vi "Read Multiple Event Registration.vi"(11 "Test Case In":refnum<class "Tests Event MessengerM.lvclass">) -> (0 "error out":errorcluster, 3 "Test Case Out":refnum<class "Tests Event MessengerM.lvclass">)   [LabVIEW 2020, in "Tests Event MessengerM.lvclass"]
uses:
  Tests Event MessengerM.lvclass
  Tests Event MessengerM.lvclass/Tests Event MessengerM.ctl
  C:/Program Files/National Instruments/LabVIEW 2026/vi.lib/Astemes/LUnit/Test Case.lvclass
  C:/Program Files/National Instruments/LabVIEW 2026/vi.lib/Astemes/LUnit/LUnit Runnable.lvclass
  D:/git/Event-MessengerM-Channel-Wire/tests/Tests Event MessengerM/Tests Event MessengerM.lvclass
  <vilib>/Astemes/LUnit/Test Case.lvclass
  4a87e2e1-9280-4bda-9c4f-14fca454df33.vi
  66c5d38c-d599-4b3c-b5fe-0ff2804ba194.vi
  4a2384a7-b9c3-4d6f-8ce3-db5ad262e870.vi
  3cda7afb-27d7-4926-bd3c-22bc82fc3959.vi
  fb264298-76b7-4d75-ae4f-a2dcca52a52e.vi
panel:
  out "Array 2":string[](array[string])
  out "Array":string[](array[string])
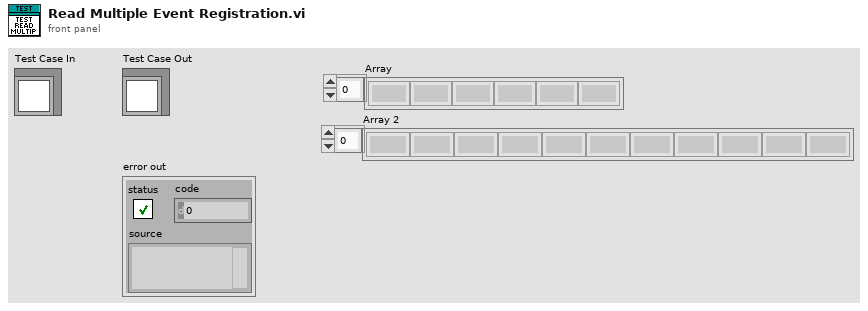
[diagram p1: front panel]
types:
  T1 = typedef "Event MessengerM-c(str,var).lvlib/))Channel.ctl" = refnum<queue>
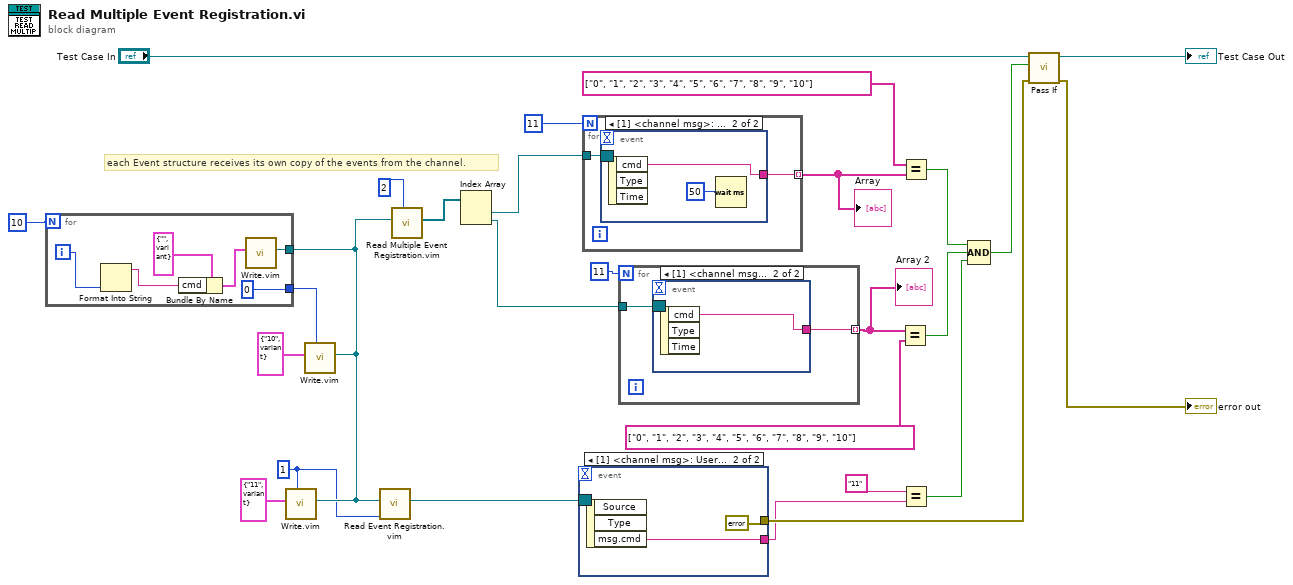
[diagram p0: block diagram]
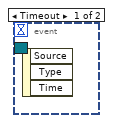
[diagram p2: hidden frame]
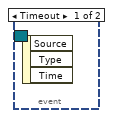
[diagram p3: hidden frame]
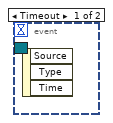
[diagram p4: hidden frame]
diagram:
  w2 = 1 ("subchannel (0)")
  # "each Event structure receives its own copy of the events from the channel."
  n1 = for {
    N: 10 -> [_]
    tunnel: [0] -> w7
    tunnel: [w28] -> w4
    i -> [w32]
    n2 = Format Into String(w32) -> (resulting string=w31:string)  [unwired: 3 in, 1 out]
    n3 = Bundle By Name(cluster=cluster{"cmd":string, "data":variant} {"cmd"="", "data"=variant} ("element"), "cmd"=w31) -> (w29:cluster{"cmd":string, "data":variant})
    n4 = call "Write.vim"("element"=w29) -> ("channel"=w28:T1)  [unwired: 9 in, 1 out]
  }
  n5 = call "Write.vim"("channel"=w4, "subchannel"=w2, "element"=cluster{"cmd":string, "data":variant} {"cmd"="11", "data"=variant}) -> ()  [unwired: 8 in, 1 out]
  n6 = call "Write.vim"("channel"=w4, "subchannel"=w7, "element"=cluster{"cmd":string, "data":variant} {"cmd"="10", "data"=variant}) -> ()  [unwired: 8 in, 1 out]
  n7 = call "Read Event Registration.vim"("subchannel"=w2, "channel"=w4) -> ("event registration refnum"=w5:refnum<event-registration>)  [unwired: 9 in]
  n8 = call "Read Multiple Event Registration.vim"("number of event structures"=u16 2, "channel in"=w4) -> ("event registration refnums"=w1:refnum<event-registration>[])  [unwired: 9 in]
  n9 = Index Array(array=w1) -> (element #1=w17:refnum<event-registration>, element #2=w16:refnum<event-registration>)  [unwired: 2 in]
  n10 = event shown="[1] <channel msg>: User Event" {
    selector: w5 -> [_ _]
    dyn-events: _ -> [_ _]
    timeout: _ -> [_ _]
    tunnel: [_ errorcluster {"status"=FALSE, "code"=0, "source"=""} ("error constant")] -> w18
    tunnel: [_ w34] -> w13
    event Timeout {
      n11 = event-data() -> ()  [unwired: 1 in, 3 out]
    }
    event User Event {
      n12 = event-data() -> ("msg.cmd"=w34:string)  [unwired: 1 in, 2 out]
    }
  }
  n13 = for {
    N: 11 -> [_]
    tunnel: w17 -> [w36]
    tunnel: [w37] -> w15 mode=indexing
    n14 = event shown="[1] <channel msg>: User Event" {
      selector: w36 -> [_ _]
      dyn-events: _ -> [_ _]
      timeout: _ -> [_ _]
      tunnel: [_ w39] -> w37
      event Timeout {
        n15 = event-data() -> ()  [unwired: 1 in, 3 out]
      }
      event User Event {
        n16 = event-data() -> ("cmd"=w39:string)  [unwired: 1 in, 2 out]
        n17 = Wait (ms)(milliseconds to wait=u32 50) -> ()  [unwired: 1 out]
      }
    }
  }
  "Array" <- w15
  n18 = for {
    N: 11 -> [_]
    tunnel: [w41] -> w14 mode=indexing
    tunnel: w16 -> [w40]
    n19 = event shown="[1] <channel msg>: User Event" {
      selector: w40 -> [_ _]
      dyn-events: _ -> [_ _]
      timeout: _ -> [_ _]
      tunnel: [_ w42] -> w41
      event Timeout {
        n20 = event-data() -> ()  [unwired: 1 in, 3 out]
      }
      event User Event {
        n21 = event-data() -> ("cmd"=w42:string)  [unwired: 1 in, 2 out]
      }
    }
  }
  "Array 2" <- w14
  n22 = Equal?(x=w14, y=string[] ["0", "1", "2", "3", "4", "5", "6", "7", "8", "9", "10"] ("Array 2")) -> (x = y?=w21:bool)
  n23 = Equal?(x=string[] ["0", "1", "2", "3", "4", "5", "6", "7", "8", "9", "10"] ("Array 2"), y=w15) -> (x = y?=w20:bool)
  n24 = Equal?(x="11", y=w13) -> (x = y?=w11:bool)
  n25 = Compound Arithmetic op=AND(w20, w21, w11) -> (w19:bool)
  n26 = call <vilib>:"Pass If.vi"("error in (no error)"=w18, "Pass?"=w19, "LUnit Test Case In"="Test Case In") -> ("error out"=→"error out":errorcluster, "LUnit Test Case Out"=→"Test Case Out":refnum<class "Tests Event MessengerM.lvclass">)  [unwired: 7 in]
